vi "RemotePanelMethods-Server_TerraNova.vi"() -> ()   [LabVIEW 2009]
doc: "This VI illustrates how to programmatically monitor and control remote front panel connections. It utilizes the new VI server properties and methods introduced in LabVIEW 7.0 to monitor connections, lock and unlock control and close connections. \nIt is used in conjunction with the Remote Panel Client.vi example. \n\nThis server VI serves as a model of how you could allow a client to only run a VI once after connecting and taking control. The following steps are performed:\n1. Starts web server.\n2. Polls for connections & control while displaying this information on the front panel.\n3. Waits until the client runs the VI once and then locks control and disconnects the client.\n\nAlso, for these examples to work, the web server must be enabled on the server machine. This VI programmatically starts the web server although you could also start it by going to the Web Server: Configuration Menu in Tools->Options."
panel:
  out "Web Server Port":u16
  out "Control":bool
  out "Connection Status":string
  # "Instructions:   \n1.  Make sure the Web Server is configured properly. This can be done from Tools>>Options in the \"Web Server\"\n     pages. The client machine needs to be given viewing and controlling abilities in the Browser Access List.\n2.  Open the Remote Panel Client.vi example that is used in conjunction with this example.\n     NOTE:This must be done in another LabVIEW of the same version since a remote panel connection\n     cannot be made from a LabVIEW to itself.\n3.  Run this VI and then follow the instructions given on the Client VI.\n4.  Monitor the connection and control status below."
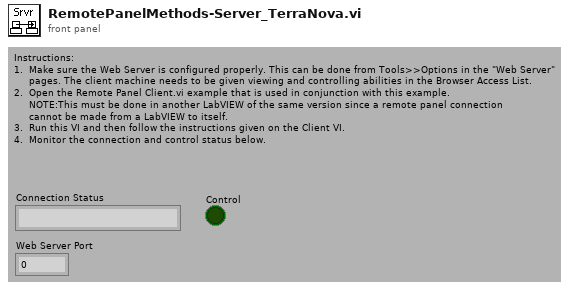
[diagram p1: front panel]
types:
  T1 = enum32{"Bad", "Idle", "Run top level", "Running"}
  T2 = typedef "LVRemotePanelConnectionsTypeDef.ctl" = cluster{"VI Name":string, "Remote":string, "UserName":string, "Port":i32, "Status":enum32{"Viewing", "Waiting For Control", "Controlling"}, "Create Time":timestamp, "Status Time":timestamp, "Control End Time":timestamp}[]
  T3 = cluster{"VI Name":string, "Remote":string, "UserName":string, "Port":i32, "Status":enum32{"Viewing", "Waiting For Control", "Controlling"}, "Create Time":timestamp, "Status Time":timestamp, "Control End Time":timestamp}
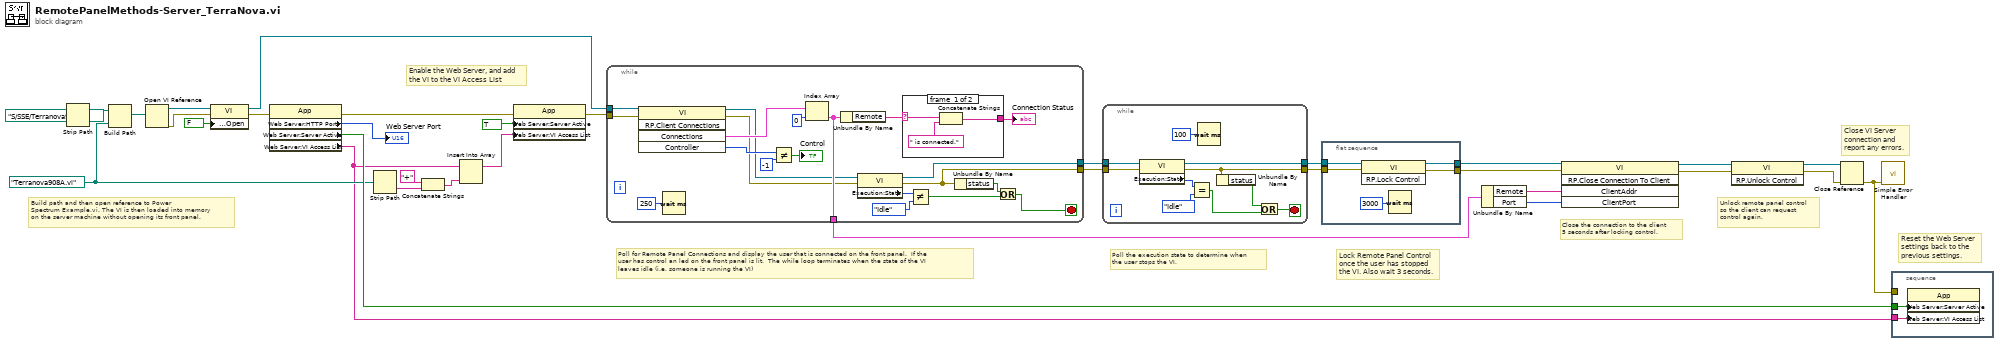
[diagram p0: block diagram]
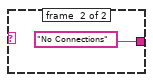
[diagram p2: hidden frame]
diagram:
  w6 = path "Terranova908A.vi"
  # "Enable the Web Server, and add\nthe VI to the VI Access List"
  # "Reset the Web Server\nsettings back to the\nprevious settings."
  # "Build path and then open reference to Power \nSpectrum Example.vi. The VI is then loaded into memory \non the server machine without opening its front panel."
  # "Close VI Server \nconnection and \nreport any errors."
  # "Unlock remote panel control\nso the client can request \ncontrol again."
  # "Close the connection to the client\n5 seconds after locking control."
  # "Lock Remote Panel Control\nonce the user has stopped\nthe VI. Also wait 3 seconds."
  # "Poll the execution state to determine when\nthe user stops the VI."
  # "Poll for Remote Panel Connections and display the user that is connected on the front panel.  If the\nuser has control an led on the front panel is lit.  The while loop terminates when the state of the VI\nleaves idle (i.e. someone is running the VI)"
  n1 = Strip Path(path=path "S:/SSE/Terranova908A/ ") -> (stripped path=w25:path)  [unwired: 1 out]
  n2 = Build Path(base path=w25, name or relative path=w6) -> (appended path=w28:path)
  n3 = Open VI Reference(vi path=w28) -> (vi reference=w27:refnum<vi>, error out=w26:errorcluster)  [unwired: 5 in]
  n4 = property class="VI"(reference=w27, error in=w26, "Front Panel Window:Open"=FALSE) -> (reference out=w13:refnum<vi>, error out=w11:errorcluster)
  n5 = property class="App"(error in=w11) -> (error out=w10:errorcluster, "Web Server:HTTP Port"=→"Web Server Port":u16, "Web Server:Server Active"=w7:bool, "Web Server:VI Access List"=w2:string[])  [unwired: 1 in, 1 out]
  n6 = Strip Path(path=w6) -> (name=w5:string)  [unwired: 1 out]
  n7 = Concatenate Strings("+" ("string"), w5) -> (w4:string)
  n8 = Insert Into Array(array=w2, new element=w4) -> (w1:string[])  [unwired: 1 in]
  n9 = property class="App"(error in=w10, "Web Server:Server Active"=TRUE, "Web Server:VI Access List"=w1) -> (error out=w14:errorcluster)  [unwired: 1 in, 1 out]
  n10 = while {
    tunnel: [w45] -> w19
    tunnel: w13 -> [w44]
    tunnel: w14 -> [w43]
    tunnel: [w35] -> w24
    tunnel: [w34] -> w23
    stop <- w47 stop-if-true
    n11 = invoke class="VI" method="RP.Client Connections"(reference=w44, error in=w43) -> (reference out=w36:refnum<vi>, error out=w39:errorcluster, "Connections"=w52:T2, "Controller"=w49:i32)  [unwired: 3 in, 1 out]
    n12 = Wait (ms)(milliseconds to wait=u32 250) -> ()  [unwired: 1 out]
    n13 = Not Equal?(x=w49, y=-1) -> (x != y?=→"Control":bool)
    n14 = Index Array(array=w52, index=0) -> (element=w45:T3)
    n15 = Unbundle By Name(w45) -> ("Remote"=w50:string)
    n16 = property class="VI"(reference=w36, error in=w39) -> (reference out=w34:refnum<vi>, error out=w35:errorcluster, "Execution:State"=w41:T1)
    n17 = case shown="\"\"" w50 {
      selector: w50 -> [w56 _]
      tunnel: [w54 "No Connections"] -> w46
      frame #0 {
        n18 = Concatenate Strings(w56, " is connected." ("string")) -> (w54:string)
      }
      frame #1 {
      }
    }
    "Connection Status" <- w46
    n19 = Not Equal?(x=w41, y=T1."Idle" ("Execution:State")) -> (x != y?=w38:bool)
    n20 = Unbundle By Name(w35) -> ("status"=w37:bool)
    n21 = Or(x=w37, y=w38) -> (x .or. y?=w47:bool)
  }
  n22 = while {
    tunnel: w24 -> [w67]
    tunnel: w23 -> [w65]
    tunnel: [w61] -> w22
    tunnel: [w58] -> w18
    stop <- w62 stop-if-true
    n23 = property class="VI"(reference=w65, error in=w67) -> (reference out=w58:refnum<vi>, error out=w61:errorcluster, "Execution:State"=w64:T1)
    n24 = Equal?(x=w64, y=T1."Idle" ("Execution:State")) -> (x = y?=w59:bool)
    n25 = Wait (ms)(milliseconds to wait=u32 100) -> ()  [unwired: 1 out]
    n26 = Unbundle By Name(w61) -> ("status"=w60:bool)
    n27 = Or(x=w60, y=w59) -> (x .or. y?=w62:bool)
  }
  n28 = flat-sequence {
    tunnel: w22 -> [w72]
    tunnel: [w70] -> w21
    tunnel: [w69] -> w20
    tunnel: w18 -> [w68]
    frame #0 {
      n29 = invoke class="VI" method="RP.Lock Control"(reference=w68, error in=w72) -> (reference out=w69:refnum<vi>, error out=w70:errorcluster)  [unwired: 1 in, 1 out]
      n30 = Wait (ms)(milliseconds to wait=u32 3000) -> ()  [unwired: 1 out]
    }
  }
  n31 = Unbundle By Name(w19) -> ("Remote"=w16:string, "Port"=w15:i32)
  n32 = invoke class="VI" method="RP.Close Connection To Client"(reference=w20, error in=w21, "ClientAddr"=w16, "ClientPort"=w15) -> (reference out=w32:refnum<vi>, error out=w33:errorcluster)  [unwired: 1 in, 3 out]
  n33 = invoke class="VI" method="RP.Unlock Control"(reference=w32, error in=w33) -> (reference out=w31:refnum<vi>, error out=w30:errorcluster)  [unwired: 1 in, 1 out]
  n34 = Close Reference(reference=w31, error in (no error)=w30) -> (error out=w8:errorcluster)
  n35 = call <vilib>:"Simple Error Handler.vi"("error in (no error)"=w8) -> ()  [unwired: 4 in, 5 out]
  n36 = stacked-sequence {
    tunnel: w8 -> [_]
    tunnel: w7 -> [w74]
    tunnel: w2 -> [w73]
    frame #0 {
      n37 = property class="App"("Web Server:Server Active"=w74, "Web Server:VI Access List"=w73) -> ()  [unwired: 2 in, 2 out]
    }
  }
